vi "Check_EnFlo_Tunnel_Cond.vi"() -> (0 "Status Cluster":T1, 1 "Heaters On?":bool)   [LabVIEW 2010]
uses:
  Anemometry/Anemometry Sub Vis/Gen Trav/Status_Cluster.ctl
  Anemometry/Anemometry Sub Vis/Gen Trav/Multi_Run_Status.ctl
  Anemometry/Anemometry Sub Vis/Controls/In_Range.ctl
  Anemometry/Anemometry Sub Vis/Globals/Meas_global.vi
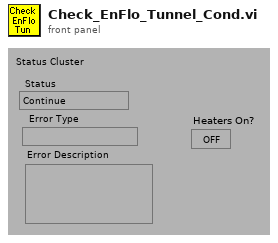
[diagram p1: front panel]
types:
  T1 = typedef "Status_Cluster.ctl" = cluster{"Status":T2, "Error Type":string, "Error Description":string}
  T2 = typedef "Multi_Run_Status.ctl" = enum16{"Continue", "Jump to Next Point", "Jump to Next Row", "Jump To Fall Back", "Terminate Run"}
  T3 = typedef "In_Range.ctl" = enum16{"%", "±", "% & ±"}
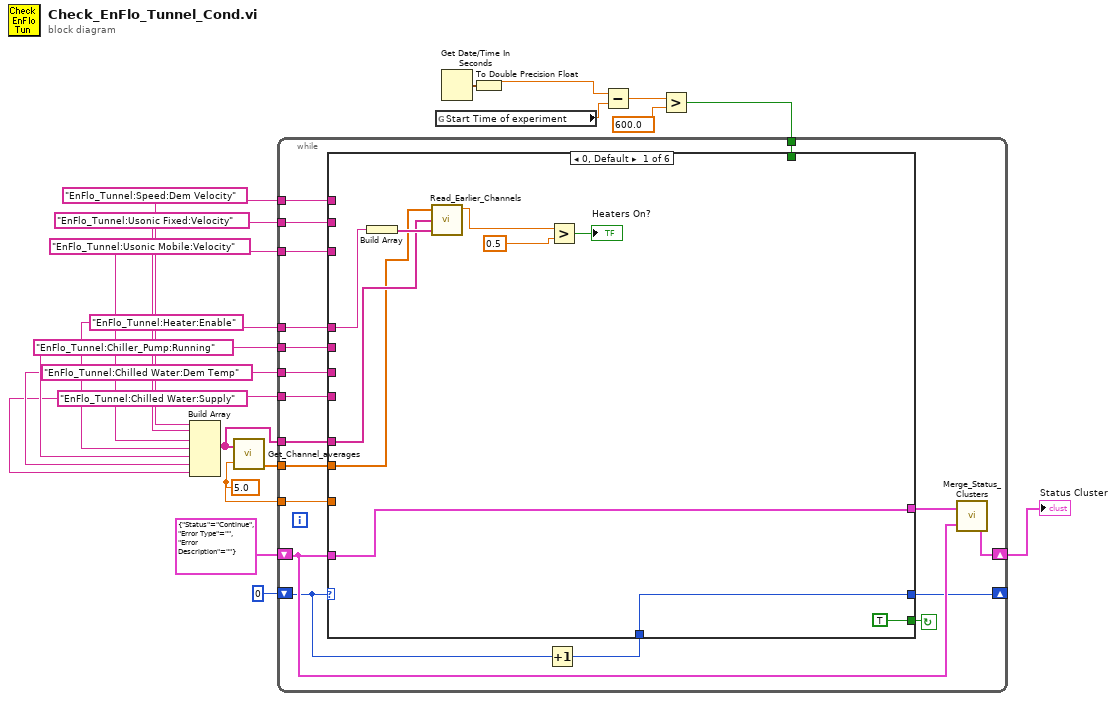
[diagram p0: block diagram]
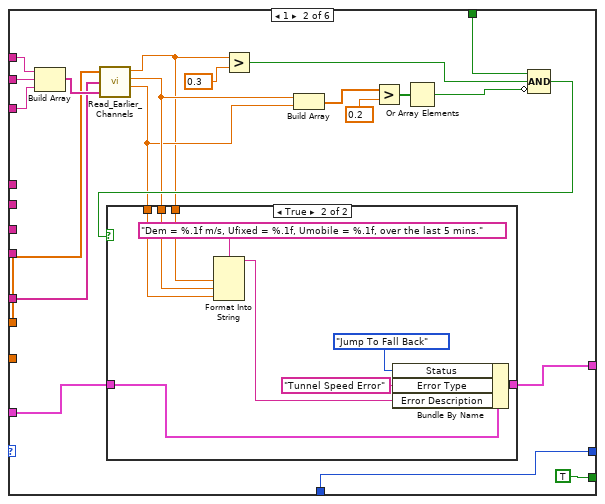
[diagram p2: hidden frame]
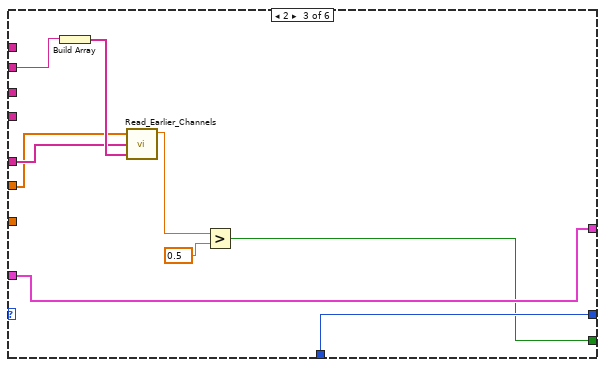
[diagram p4: hidden frame]
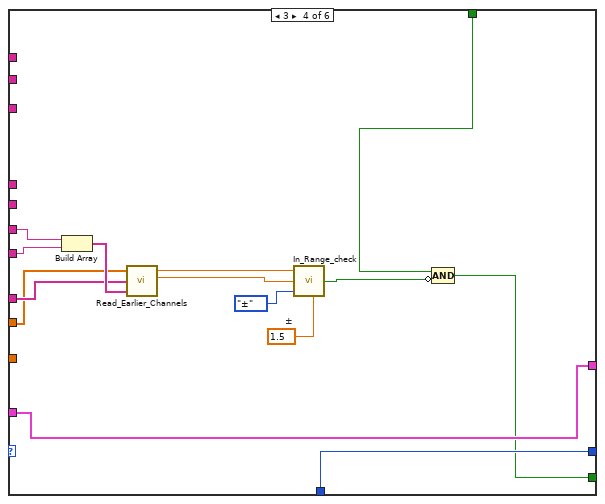
[diagram p5: hidden frame]
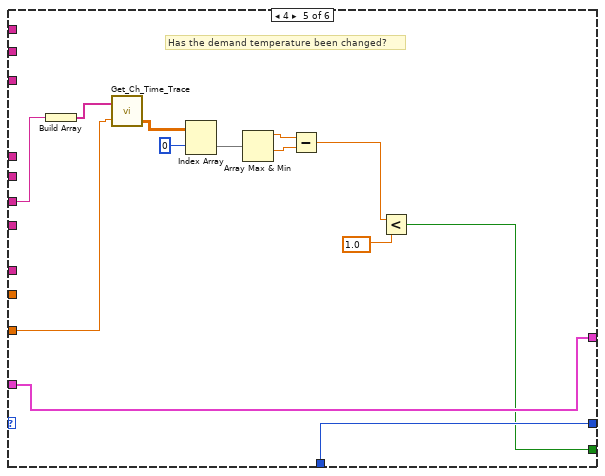
[diagram p6: hidden frame]
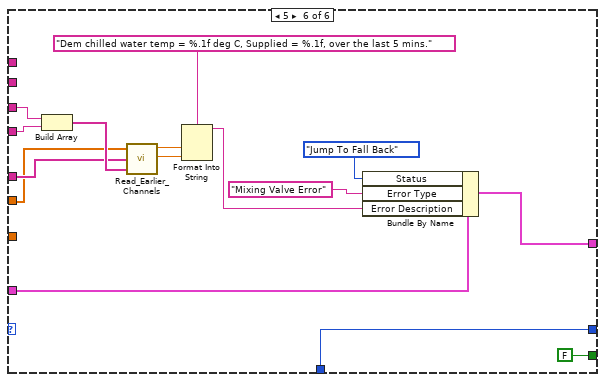
[diagram p7: hidden frame]
diagram:
  w8 = "EnFlo_Tunnel:Chilled Water:Supply"
  w9 = "EnFlo_Tunnel:Chilled Water:Dem Temp"
  w10 = "EnFlo_Tunnel:Chiller_Pump:Running"
  w15 = "EnFlo_Tunnel:Heater:Enable"
  w1 = 5.0 ("Averaging time (mins)")
  w18 = "EnFlo_Tunnel:Speed:Dem Velocity"
  w17 = "EnFlo_Tunnel:Usonic Fixed:Velocity"
  w16 = "EnFlo_Tunnel:Usonic Mobile:Velocity"
  n1 = Build Array(w18, w17, w16, w15, w10, w9, w8) -> (w12:string[])
  n2 = call "Get_Channel_averages.vi"("Desired Ch Names"=w12, "Averaging time (mins)"=w1) -> ("number"=w19:dbl[])  [unwired: 1 in, 2 out]
  n3 = global read "Meas_global.vi" "Start Time of experiment"() -> (w5:dbl)
  n4 = Get Date/Time In Seconds() -> (seconds since 1Jan1904=w2:timestamp)
  n5 = To Double Precision Float(number=w2) -> (double precision float=w4:dbl)
  n6 = Subtract(x=w4, y=w5) -> (x-y=w6:dbl)
  n7 = Greater?(x=w6, y=600.0) -> (0:w3:bool)
  n8 = while {
    tunnel: w3 -> [w21]
    tunnel: w8 -> [w22]
    tunnel: w9 -> [w23]
    tunnel: w10 -> [w24]
    shift-left: 0 -> [w27]
    shift-right: [w26] -> _
    tunnel: w15 -> [w31]
    tunnel: w16 -> [w32]
    tunnel: w17 -> [w33]
    tunnel: w18 -> [w34]
    tunnel: w12 -> [w35]
    tunnel: w19 -> [w36]
    shift-left: T1 {"Status"=enum."Continue", "Error Type"="", "Error Description"=""} ("Status Cluster In") -> [w29]
    shift-right: [w28] -> w14
    tunnel: w1 -> [w20]
    stop <- w37 continue-if-true
    n9 = Increment(x=w27) -> (x+1=w25:i32)
    n10 = case shown="0, Default" w27 {
      tunnel: [TRUE TRUE w80 w88 w110 FALSE] -> w37
      tunnel: w36 -> [w42 w58 w84 w98 _ w127]
      tunnel: w35 -> [w43 w59 w85 w99 _ w128]
      tunnel: w34 -> [_ w63 _ _ _ _]
      tunnel: w33 -> [_ w62 _ _ _ _]
      tunnel: w32 -> [_ w61 _ _ _ _]
      tunnel: w29 -> [w47 w67 w87 w101 w114 w116]
      tunnel: [w47 w65 w87 w101 w114 w115] -> w30
      tunnel: w31 -> [w40 _ _ _ _ _]
      tunnel: w25 -> [w41 w49 w83 w97 w113 w126]
      tunnel: [w41 w49 w83 w97 w113 w126] -> w26
      tunnel: w24 -> [_ _ w82 _ _ _]
      tunnel: w23 -> [_ _ _ w96 w109 w124]
      tunnel: w22 -> [_ _ _ w95 _ w125]
      tunnel: w21 -> [_ w48 _ w89 _ _]
      tunnel: w20 -> [_ _ _ _ w107 _]
      frame 0, Default {
        n11 = Build Array(w40) -> (w44:string[])
        n12 = call "Read_Earlier_Channels.vi"("Present scan array"=w42, "Ch names"=w43, "Desired Channels"=w44) -> ("Index 0"=w39:dbl)  [unwired: 5 out]
        n13 = Greater?(x=w39, y=0.5) -> (0:→"Heaters On?":bool)
      }
      frame 1 {
        n14 = Build Array(w63, w62, w61) -> (w60:string[])
        n15 = call "Read_Earlier_Channels.vi"("Present scan array"=w58, "Ch names"=w59, "Desired Channels"=w60) -> ("Index 0"=w55:dbl, "Index 1"=w57:dbl, "Index 2"=w56:dbl)  [unwired: 3 out]
        n16 = Greater?(x=w55, y=0.3) -> (0:w50:bool)
        n17 = Build Array(w57, w56) -> (w53:dbl[])
        n18 = Greater?(x=w53, y=0.2) -> (0:w51:bool[])
        n19 = Or Array Elements(Boolean array=w51) -> (logical OR=w66:bool)
        n20 = Compound Arithmetic op=AND(w48, w50, invert w66) -> (w64:bool)
        n21 = case shown="True" w64 {
          tunnel: [w69 w77] -> w65
          tunnel: w67 -> [w69 w78]
          tunnel: w55 -> [_ w72]
          tunnel: w57 -> [_ w71]
          tunnel: w56 -> [_ w70]
          frame False {
          }
          frame True {
            n22 = Format Into String(format string="Dem = %.1f m/s, Ufixed = %.1f, Umobile = %.1f, over the last 5 mins." ("Format String"), w72, w71, w70) -> (resulting string=w73:string)  [unwired: 2 in, 1 out]
            n23 = Bundle By Name(cluster=w78, "Status"=Multi_Run_Status."Jump To Fall Back", "Error Type"="Tunnel Speed Error" ("Bundle Element"), "Error Description"=w73) -> (w77:T1)
          }
        }
      }
      frame 2 {
        n24 = Build Array(w82) -> (w86:string[])
        n25 = call "Read_Earlier_Channels.vi"("Present scan array"=w84, "Ch names"=w85, "Desired Channels"=w86) -> ("Index 0"=w79:dbl)  [unwired: 5 out]
        n26 = Greater?(x=w79, y=0.5) -> (0:w80:bool)
      }
      frame 3 {
        w92 = 1.5  # ±
        n27 = Build Array(w96, w95) -> (w100:string[])
        n28 = call "Read_Earlier_Channels.vi"("Present scan array"=w98, "Ch names"=w99, "Desired Channels"=w100) -> ("Index 0"=w94:dbl, "Index 1"=w93:dbl)  [unwired: 4 out]
        n29 = call "In_Range_check.vi"("±"=w92, "Mode"=In_Range."±", "Value"=w93, "Setpoint"=w94) -> ("In Range"=w90:bool)  [unwired: 1 in, 2 out]
        n30 = Compound Arithmetic op=AND(w89, invert w90) -> (w88:bool)
      }
      frame 4 {
        # "Has the demand temperature been changed?"
        n31 = Build Array(w109) -> (w108:string[])
        n32 = call "Get_Ch_Time_Trace.vi"("Desired Ch Names"=w108, "History Length (mins)"=w107) -> ("Output array"=w106:dbl[][])  [unwired: 2 out]
        n33 = Index Array(array=w106, index (row)=0 ("Index")) -> (element=w105:dbl[])  [unwired: 1 in]
        n34 = Array Max & Min(array=w105) -> (max value=w104:dbl, min value=w103:dbl)  [unwired: 2 out]
        n35 = Subtract(x=w104, y=w103) -> (x-y=w102:dbl)
        n36 = Less?(x=w102, y=1.0) -> (x < y?=w110:bool)
      }
      frame 5 {
        n37 = Build Array(w124, w125) -> (w129:string[])
        n38 = call "Read_Earlier_Channels.vi"("Present scan array"=w127, "Ch names"=w128, "Desired Channels"=w129) -> ("Index 0"=w118:dbl, "Index 1"=w117:dbl)  [unwired: 4 out]
        n39 = Format Into String(format string="Dem chilled water temp = %.1f deg C, Supplied = %.1f, over the last 5 mins." ("Format String"), w118, w117) -> (resulting string=w119:string)  [unwired: 2 in, 1 out]
        n40 = Bundle By Name(cluster=w116, "Status"=Multi_Run_Status."Jump To Fall Back", "Error Type"="Mixing Valve Error" ("Bundle Element"), "Error Description"=w119) -> (w115:T1)
      }
    }
    n41 = call "Merge_Status_Clusters.vi"("Status Cluster 2"=w29, "Status Cluster 1"=w30) -> ("Status Cluster Out"=w28:T1)
  }
  "Status Cluster" <- w14
